vi "SRV_Wait (ms)+.vi"(7 "milliseconds to wait":u32, 11 "error in (no error)":errorcluster) -> (8 "millisecond timer value":u32, 15 "error out":errorcluster)   [LabVIEW 2014]
doc: "Waits the specified number of milliseconds and returns the value of the millisecond timer. If there is an input error, the millisecond timer value is returned, but the VI does not wait.\n\nThis VI is an enhancement of the \"Wait (ms)\" function, adding error inputs and outputs.\n\n\nAuthor: Mike Schultz"
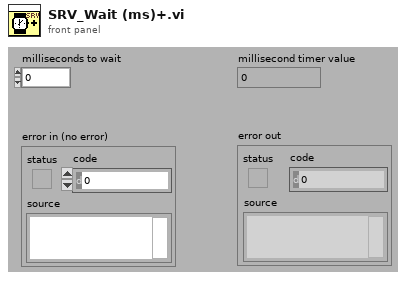
[diagram p1: front panel]
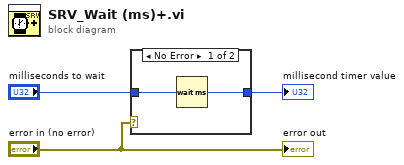
[diagram p0: block diagram]
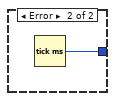
[diagram p2: hidden frame]
diagram:
  n1 = case shown="No Error" "error in (no error)" {
    tunnel: "milliseconds to wait" -> [w5 _]
    tunnel: [w4 w6] -> w2
    frame No Error {
      n2 = Wait (ms)(milliseconds to wait=w5) -> (millisecond timer value=w4:u32)
    }
    frame Error {
      n3 = Tick Count (ms)() -> (millisecond timer value=w6:u32)
    }
  }
  "millisecond timer value" <- w2
  "error out" <- "error in (no error)"
